vi "Set SPAN Component Tables.vi"(4 "EPA Optionsfeld":T2=enum."Rohwert", 6 "Polynom-Ordnung":T1, 8 "error in (no error)":errorcluster caption="Fehler (Eingang, kein Fehler)", 9 "Gaskomponente":T9, 10 "postprocess":bool, 11 "Tabellenref.":refnum<vi>) -> (0 "error out":errorcluster caption="Fehler (Ausgang)", 1 "EPA Ausgangs-Cluster":T4, 2 "LIN Ausgangs-Cluster":T3, 3 "Daten Aufzeichnen Ausgangs-Cluster":T6, 5 "Aktiv EPA":T7, 7 "Aktiv LIN":bool[](array[boolean]))   [LabVIEW 2020, in "Linearisierung v2.lvlib" / "SpanEinstellungen.lvlib"]
uses:
  SpanEinstellungen.lvlib
  Visualisierungs Elemente/Auswahlfeld.ctl
  AktivArray.ctl
  AktivButton.ctl
  Ausgabetabelle.ctl
  EPA Optionsfeld.ctl
  Auswahl Polynom Ordnung.ctl
  Aktion Lin Daten aufarbeiten.ctl
  EPA1065-307/Aktion FGV Auswertung sammeln.ctl
  Linearisierung v2.lvlib
  EPA1065-307/Linearity verification 1065-307.lvlib
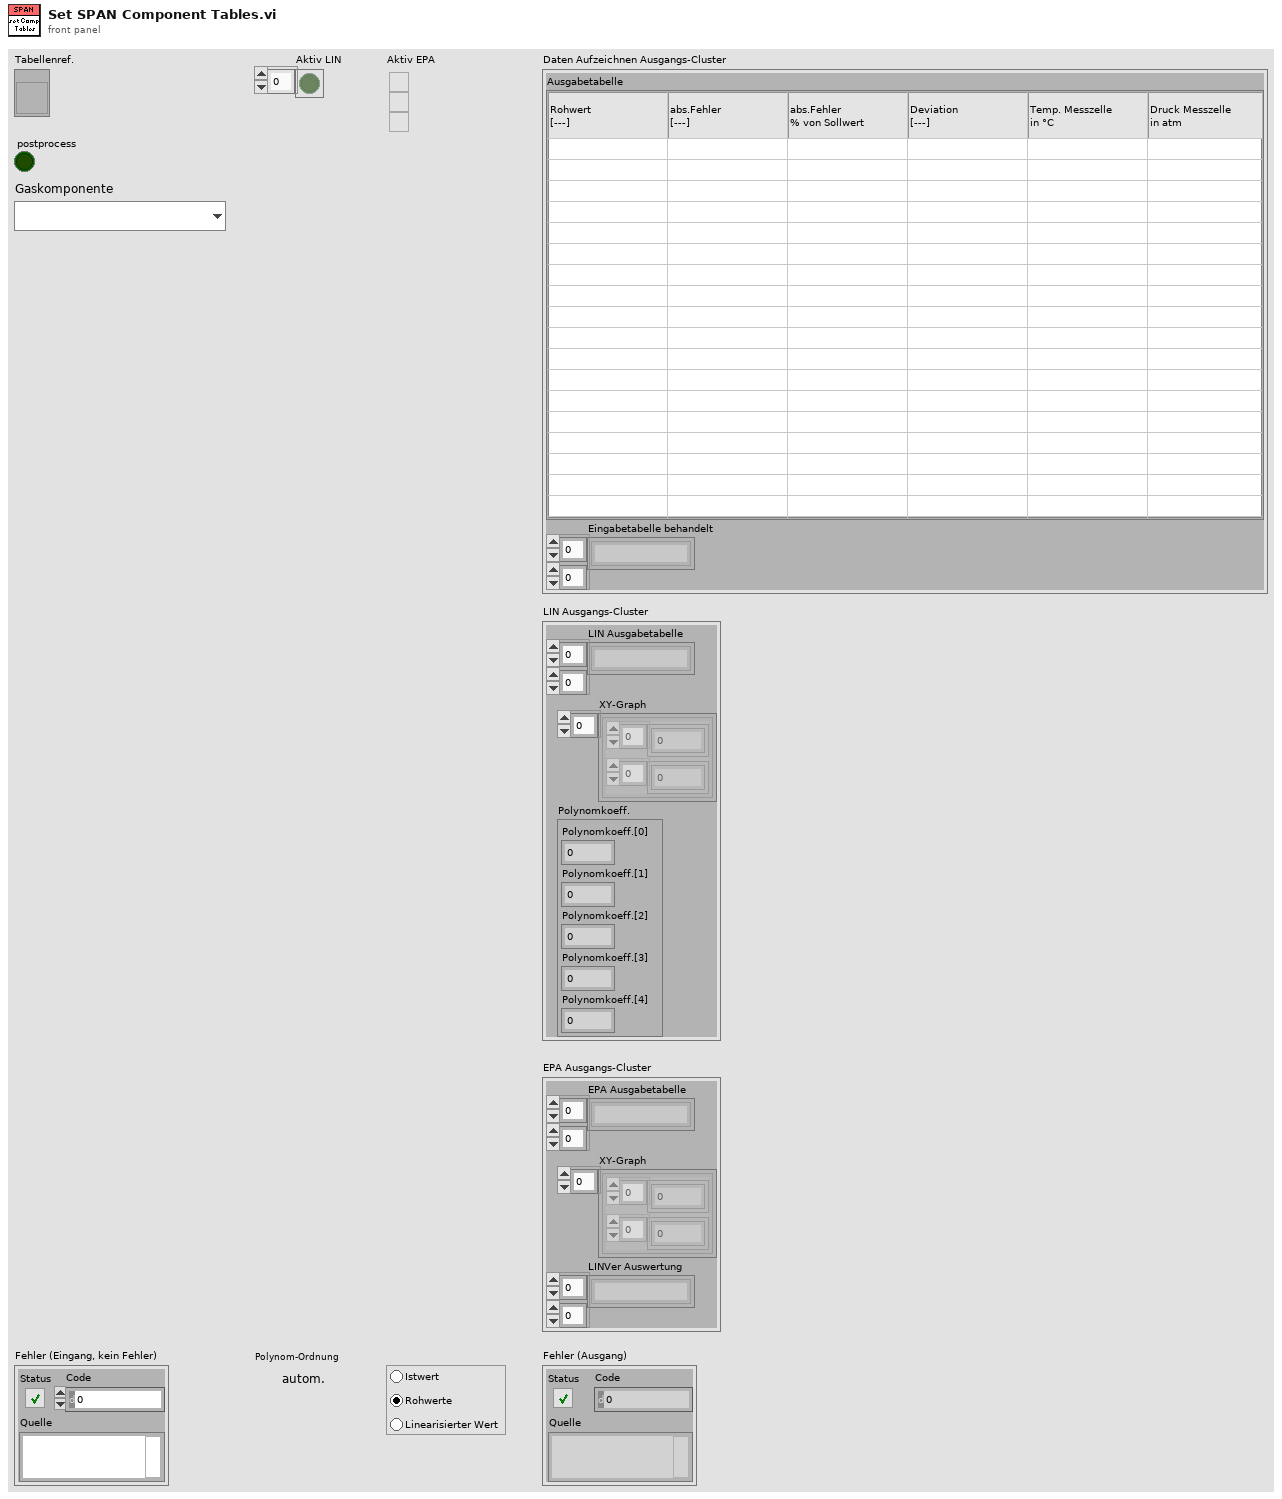
[diagram p1: front panel]
types:
  T1 = typedef "Linearisierung v2.lvlib/Auswahl Polynom Ordnung.ctl" = enum16{"autom.", "raw", "actual", "1", "2", "3", "4"}
  T2 = typedef "Linearisierung v2.lvlib/EPA Optionsfeld.ctl" = enum32{"Istwert", "Rohwert", "Linearisierter Wert"}
  T3 = cluster{"LIN Ausgabetabelle ":string[][], "XY-Graph":cluster{dbl[], dbl[]}[], "Polynomkoeff.":cluster{"Polynomkoeff.[0]":sgl, "Polynomkoeff.[1]":sgl, "Polynomkoeff.[2]":sgl, "Polynomkoeff.[3]":sgl, "Polynomkoeff.[4]":sgl}}
  T4 = cluster{"EPA Ausgabetabelle ":string[][], "XY-Graph":cluster{dbl[], dbl[]}[], "LINVer Auswertung":string[][]}
  T5 = typedef "Linearisierung v2.lvlib/Ausgabetabelle.ctl" = string[][]
  T6 = cluster{"Ausgabetabelle":T5, "Eingabetabelle behandelt":string[][]}
  T7 = typedef "Linearisierung v2.lvlib/AktivArray.ctl" = T8[]
  T8 = typedef "Linearisierung v2.lvlib/AktivButton.ctl" = bool
  T9 = typedef "Auswahlfeld.ctl" = u16
  T10 = typedef "Linearisierung v2.lvlib/Aktion Lin Daten aufarbeiten.ctl" = enum16{"lesen", "Protkolldaten", "speichern", "laden", "EPA auswerten", "Tabelle schreiben", "Lin auswerten", "Tab init", "Stufentabelle", "EPA aktiviert", "Nachbehandlung laden", "Tabelle löschen", "Istwerte löschen", "Zeile löschen", "Zeile einfügen", "LIN aktiviert", "LIN/EPA aktiv laden", "EGAK Tab", "LIN übernehmen", "Tab init ohne Stufen"}
  T11 = typedef "Linearisierung v2.lvlib/Linearity verification 1065-307.lvlib/Aktion FGV Auswertung sammeln.ctl" = enum16{"lesen", "Auswertung", "löschen"}
  T12 = typedef "Linearisierung v2.lvlib/Eingabetabelle.ctl" = string[][]
  T13 = typedef "Linearisierung v2.lvlib/Lin-Polynom Daten.ctl" = cluster{"Messgerät":string, "Kalibrator (Gasteiler)":string, "Bearbeiter/in":string, "Komponente":string, "Zeitstempel":timestamp, "F_max gefordert (%)":sgl, "F_max in %":sgl, "F_max in ppm":sgl, "Vorschlag Ordnung":i32, "Polynom OK":bool, "Polynomkoeff.":dbl[], "Prüfgas Konzentration":dbl, "Pfad EPA":string, "Pfad_LIN":string, "Gasnummer:":u8, "Komponentenauswahl":T14, "Verdünnungsgas":T15, "Zeitdauer Stufe":T16, "Anzahl Stufen":T16, "F_max in % EPA":sgl, "F_max in ppm EPA":sgl, "F_max in % LIN":sgl, "F_max in ppm LIN":sgl, "Punkte umkehren":bool, "EPA Optionsfeld":T2, "Autolin Hovacal":T17, "Spanfactors":sgl[], "Kalibrierauswahl":T18, "Conditions:":T19, "Gasflaschen Nr.:":string, "Bottle Accuracy":dbl, "Konfig Gasflasche":T20, "Gasflasche":T21, "HovaCAL Flow AutoLin":T22, "MFC Output":T23, "Gas Ablaufdatum":timestamp, "Lin Modus":T24, "zusätzliche Zeitdauer Erster Punkt":sgl, "Offsets":sgl[]}
  T14 = typedef "Linearisierung v2.lvlib/KomponentenArray.ctl" = cluster{"Komponente:":T9, "Konzentration":dbl}[]
  T15 = typedef "Linearisierung v2.lvlib/Gasteiler.lvlib/Prüfgas in.ctl" = u16
  T16 = typedef "Zahlen-Eingabefeld.ctl" = sgl
  T17 = typedef "Linearisierung v2.lvlib/Gasteiler.lvlib/HovaCal.lvlib/AutoLin Hovacal.ctl" = enum32{"Keine Auswahl", "Optionsauswahl 1", "Optionsauswahl 2"}
  T18 = typedef "Linearisierung v2.lvlib/Kalibrieroption.ctl" = u16
  T19 = typedef "Linearisierung v2.lvlib/Linearity verification 1065-307.lvlib/Condition.ctl" = u16
  T20 = typedef "System Einstellungen V2.lvlib/Konfig Gasflasche.ctl" = bool
  T21 = typedef "System Einstellungen V2.lvlib/Gasflasche Auswahl.ctl" = u16
  T22 = typedef "Linearisierung v2.lvlib/Gasteiler.lvlib/HovaCAL_Interface.lvlib/Controls.lvlib/Flow Einstellung.ctl" = cluster{"HovaCAL Flow Input Cluster":dbl}
  T23 = typedef "Linearisierung v2.lvlib/Gasteiler.lvlib/HovaCAL_Interface.lvlib/Controls.lvlib/Pump state.ctl" = cluster{"Run":bool}
  T24 = typedef "CalGas Aufschaltung.lvlib/Lin Modus.ctl" = u16
  T25 = cluster{"Polynomkoeff.[0]":dbl, "Polynomkoeff.[1]":dbl, "Polynomkoeff.[2]":dbl, "Polynomkoeff.[3]":dbl, "Polynomkoeff.[4]":dbl}
  T26 = cluster{"LIN Ausgabetabelle ":string[][], "XY-Graph":cluster{dbl[], dbl[]}[], "Polynomkoeff.":cluster{"Polynomkoeff.[0]":dbl, "Polynomkoeff.[1]":dbl, "Polynomkoeff.[2]":dbl, "Polynomkoeff.[3]":dbl, "Polynomkoeff.[4]":dbl}}
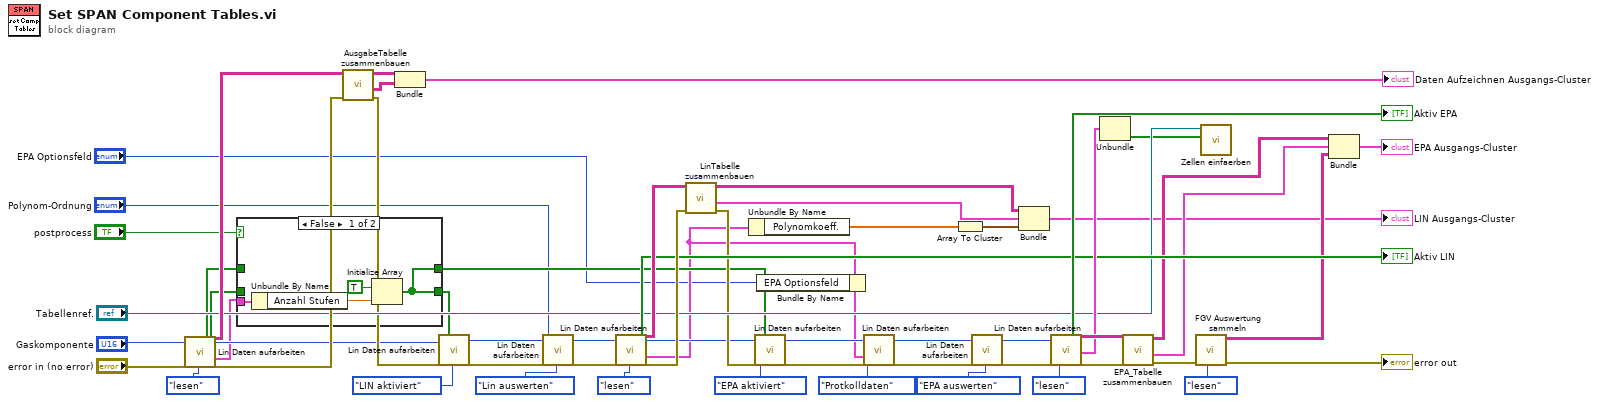
[diagram p0: block diagram]
diagram:
  n1 = call "Lin Daten aufarbeiten.vi"("Index (Seite)"="Gaskomponente", "error in (no error)"="error in (no error)", "Aktionen"=Aktion_Lin_Daten_aufarbeiten."lesen") -> ("Aktiv EPA"=w11:T7, "Aktiv LIN"=w10:bool[], "Eingabetabelle"=w60:T12, "Index (Seite) out"=w17:i32, "Lin-Polynom"=w15:T13, "error out"=w42:errorcluster)  [unwired: 14 in, 5 out]
  n2 = case shown="False" "postprocess" {
    tunnel: w15 -> [w64 _]
    tunnel: [w61 w65] -> w14
    tunnel: [w61 w66] -> w12
    tunnel: w11 -> [_ w66]
    tunnel: w10 -> [_ w65]
    frame False {
      n3 = Unbundle By Name(w64) -> ("Anzahl Stufen"=w62:T16)
      n4 = Initialize Array(TRUE, w62) -> (w61:bool[])
    }
    frame True {
    }
  }
  n5 = call "AusgabeTabelle zusammenbauen.vi"("error in (no error)"=w42, "Eingabetabelle"=w60) -> ("error out"=w19:errorcluster, "Eingabetabelle behandelt"=w35:string[][], "Ausgabetabelle"=w36:T5)  [unwired: 7 in]
  n6 = Bundle("Ausgabetabelle"=w36, "Eingabetabelle behandelt"=w35) -> (→"Daten Aufzeichnen Ausgangs-Cluster":T6)  [unwired: 1 in]
  n7 = call "Lin Daten aufarbeiten.vi"("Index (Seite)"=w17, "error in (no error)"=w19, "Aktiv"=w14, "Aktionen"=Aktion_Lin_Daten_aufarbeiten."LIN aktiviert") -> ("Index (Seite) out"=w21:i32, "error out"=w20:errorcluster)  [unwired: 13 in, 9 out]
  n8 = call "Lin Daten aufarbeiten.vi"("Index (Seite)"=w21, "error in (no error)"=w20, "Polynom-Ordnung"="Polynom-Ordnung", "Aktionen"=Aktion_Lin_Daten_aufarbeiten."Lin auswerten") -> ("Index (Seite) out"=w23:i32, "error out"=w47:errorcluster)  [unwired: 13 in, 9 out]
  n9 = call "Lin Daten aufarbeiten.vi"("Index (Seite)"=w23, "error in (no error)"=w47, "Aktionen"=Aktion_Lin_Daten_aufarbeiten."lesen") -> ("Aktiv LIN"=→"Aktiv LIN":bool[], "Eingabetabelle"=w45:T12, "Index (Seite) out"=w16:i32, "Lin-Polynom"=w4:T13, "error out"=w46:errorcluster)  [unwired: 14 in, 6 out]
  n10 = call "LinTabelle zusammenbauen.vi"("error in (no error)"=w46, "Eingabetabelle"=w45) -> ("error out"=w24:errorcluster, "XY-Graph"=w26:cluster{dbl[], dbl[]}[], "LIN Ausgabetabelle"=w27:string[][])  [unwired: 6 in, 1 out]
  n11 = Unbundle By Name(w4) -> ("Polynomkoeff."=w44:dbl[])
  n12 = call "Lin Daten aufarbeiten.vi"("Index (Seite)"=w16, "error in (no error)"=w24, "Aktiv"=w12, "Aktionen"=Aktion_Lin_Daten_aufarbeiten."EPA aktiviert") -> ("Index (Seite) out"=w7:i32, "error out"=w5:errorcluster)  [unwired: 13 in, 9 out]
  n13 = Bundle By Name(cluster=w4, "EPA Optionsfeld"="EPA Optionsfeld") -> (w3:T13)
  n14 = call "Lin Daten aufarbeiten.vi"("Index (Seite)"=w7, "Lin-Polynom"=w3, "error in (no error)"=w5, "Aktionen"=Aktion_Lin_Daten_aufarbeiten."Protkolldaten") -> ("Index (Seite) out"=w8:i32, "error out"=w6:errorcluster)  [unwired: 13 in, 9 out]
  n15 = Array To Cluster(array=w44) -> (cluster=w30:T25)
  n16 = call "Lin Daten aufarbeiten.vi"("Index (Seite)"=w8, "error in (no error)"=w6, "Aktionen"=Aktion_Lin_Daten_aufarbeiten."EPA auswerten") -> ("Index (Seite) out"=w56:i32, "error out"=w55:errorcluster)  [unwired: 14 in, 9 out]
  n17 = Bundle("LIN Ausgabetabelle"=w27, "XY-Graph"=w26, "Polynomkoeff."=w30) -> (→"LIN Ausgangs-Cluster":T26)  [unwired: 1 in]
  n18 = call "Lin Daten aufarbeiten.vi"("Index (Seite)"=w56, "error in (no error)"=w55, "Aktionen"=Aktion_Lin_Daten_aufarbeiten."lesen") -> ("Aktiv EPA"=→"Aktiv EPA":T7, "Eingabetabelle"=w54:T12, "EPA Auswertung"=w53:cluster{sgl[], sgl[], bool[]}, "error out"=w51:errorcluster)  [unwired: 14 in, 7 out]
  n19 = Unbundle(w53) -> (w37:bool[])  [unwired: 2 out]
  n20 = call "EPA_Tabelle zusammenbauen.vi"("error in (no error)"=w51, "Eingabetabelle"=w54) -> ("error out"=w50:errorcluster, "XY-Graph"=w32:cluster{dbl[], dbl[]}[], "EPA Ausgabetabelle"=w33:string[][])  [unwired: 7 in]
  n21 = call "FGV Auswertung sammeln.vi"("Aktion"=Aktion_FGV_Auswertung_sammeln."lesen", "error in (no error)"=w50) -> ("error out"=→"error out":errorcluster, "LINVer Auswertung"=w31:string[][])  [unwired: 7 in, 1 out]
  n22 = call "Zellen einfaerben.vi"("Färben"=w37, "Tabellenref."="Tabellenref.") -> ()  [unwired: 10 in]
  n23 = Bundle("EPA Ausgabetabelle"=w33, "XY-Graph"=w32, "LINVer Auswertung"=w31) -> (→"EPA Ausgangs-Cluster":T4)  [unwired: 1 in]
